vi "Test Real Positive Definite.vi"(0 "Input Matrix":T1) -> (1 "positive definite?":bool, 2 "error":i32)   [LabVIEW 2020, in "NI_AALPro.lvlib"]
doc: "Tests whether <B>Input Matrix</B> is a complex-conjugate symmetric and positive definite matrix. The data type you wire to the <B>Input Matrix</B> input determines the polymorphic instance to use."
uses:
  NI_AALPro.lvlib
  RealMatrix.ctl
  <resource>/lvanlys.dll
  NI_Matrix.lvlib
panel:
  # "Test Positive Definite"
  # "This VI is obsolete !!!\nYou should replace this VI in your diagram with the Test Matrix Type VI."
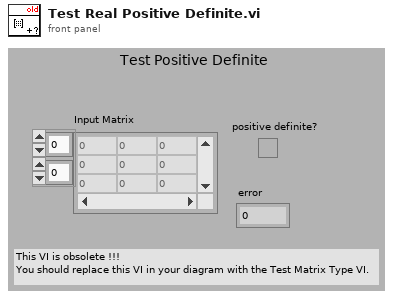
[diagram p1: front panel]
types:
  T1 = typedef "NI_Matrix.lvlib/RealMatrix.ctl" = dbl[][]
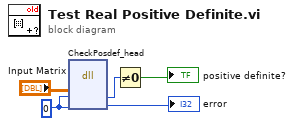
[diagram p0: block diagram]
diagram:
  w3 = 0
  n1 = dll-call lib="C:/Program Files (x86)/National Instruments/LabVIEW 2020/resource/lvanlys.*" fn="CheckPosdef_head"("Input Matrix"="Input Matrix", "output param"=w3, "output param"=w3) -> ("output param"=w2:i32, "output param"=→"error":i32)  [unwired: 5 in, 2 out]
  n2 = Not Equal To 0?(x=w2) -> (x != 0?=→"positive definite?":bool)
